vi "Get Value.vi"(8 "error in (no error)":errorcluster, 11 "Refnum Value Source in":refnum<class "Ctrl Refnum Value Source.lvclass">) -> (0 "error out":errorcluster, 2 "Value":variant, 3 "Refnum Value Source out":refnum<class "Ctrl Refnum Value Source.lvclass">)   [LabVIEW 2020, in "Composed Columns.lvlib" / "Ctrl Refnum Value Source.lvclass"]
uses:
  Ctrl Refnum Value Source.lvclass
  Ctrl Refnum Value Source.lvclass/Ctrl Refnum Value Source.ctl
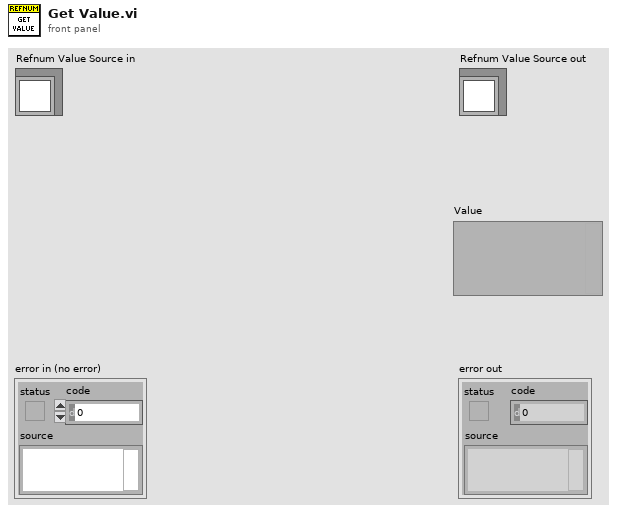
[diagram p1: front panel]
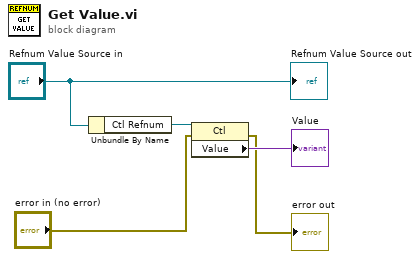
[diagram p0: block diagram]
diagram:
  n1 = Unbundle By Name("Refnum Value Source in") -> ("Ctl Refnum"=w4:refnum<vi>)
  n2 = property class="Ctl"(reference=w4, error in="error in (no error)") -> (error out=→"error out":errorcluster, "Value"=→"Value":variant)  [unwired: 1 out]
  "Refnum Value Source out" <- "Refnum Value Source in"
